vi "Example Configuration.vi"() -> ()   [LabVIEW 2010]
uses:
  C:/tf/play/labview/Tinkerforge.dll
  Tinkerforge.dll
panel:
  in  "stop":bool
  in  "uid":string="63oL6P"
  in  "port":i32=4223
  in  "host":string="localhost"
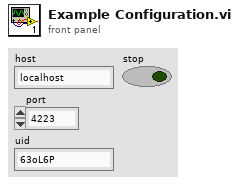
[diagram p1: front panel]
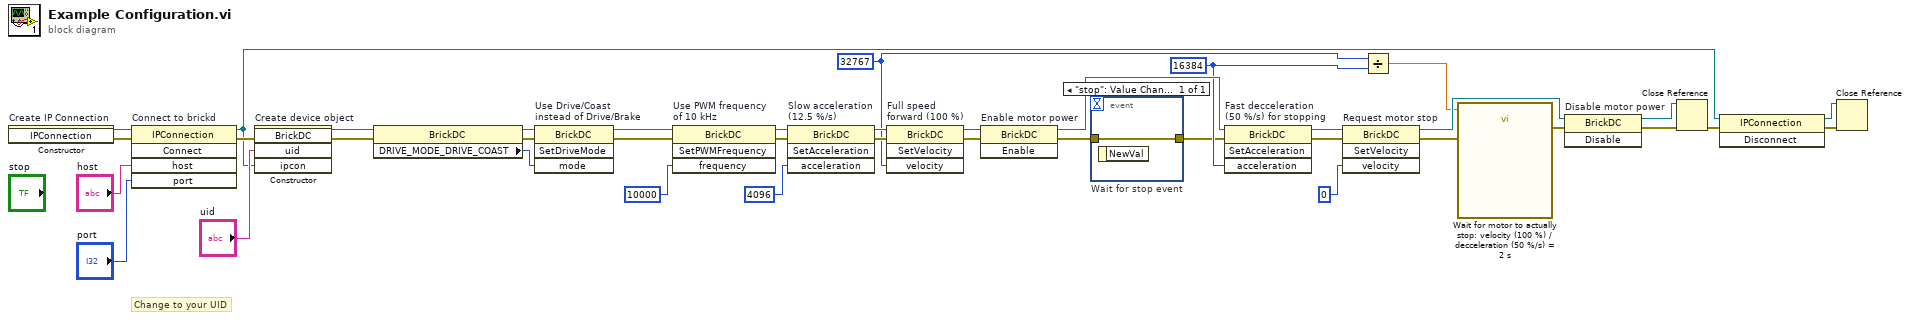
[diagram p0: block diagram]
diagram:
  w3 = 16384 ("acceleration")
  w4 = i16 32767 ("velocity")
  # "Change to your UID"
  n1 = constructor on="Create IP Connection" class="IPConnection"() -> (reference out=w39:refnum<k24>, error out=w21:errorcluster)  [unwired: 3 in, 1 out]
  n2 = invoke on="Connect to brickd" class="IPConnection" method="Connect"(reference=w39, error in=w21, "host"="host", "port"="port") -> (reference out=w32:refnum<k24>, error out=w35:errorcluster)  [unwired: 1 in, 3 out]
  n3 = constructor on="Create device object" class="BrickDC"(error in=w35, "uid"="uid", "ipcon"=w32) -> (reference out=w19:refnum<k24>, error out=w20:errorcluster)  [unwired: 2 in, 3 out]
  n4 = property class="BrickDC"(reference=w19, error in=w20) -> (reference out=w23:refnum<k24>, error out=w24:errorcluster, "DRIVE_MODE_DRIVE_COAST"=w22:u8)
  n5 = invoke on="Use Drive/Coast\ninstead of Drive/Brake" class="BrickDC" method="SetDriveMode"(reference=w23, error in=w24, "mode"=w22) -> (reference out=w18:refnum<k24>, error out=w17:errorcluster)  [unwired: 1 in, 2 out]
  n6 = invoke on="Use PWM frequency\nof 10 kHz" class="BrickDC" method="SetPWMFrequency"(reference=w18, error in=w17, "frequency"=10000 ("current")) -> (reference out=w15:refnum<k24>, error out=w16:errorcluster)  [unwired: 1 in, 2 out]
  n7 = invoke on="Slow acceleration\n(12.5 %/s)" class="BrickDC" method="SetAcceleration"(reference=w15, error in=w16, "acceleration"=4096 ("velocity")) -> (reference out=w27:refnum<k24>, error out=w28:errorcluster)  [unwired: 1 in, 2 out]
  n8 = invoke on="Full speed\nforward (100 %)" class="BrickDC" method="SetVelocity"(reference=w27, error in=w28, "velocity"=w4) -> (reference out=w25:refnum<k24>, error out=w26:errorcluster)  [unwired: 1 in, 2 out]
  n9 = invoke on="Enable motor power" class="BrickDC" method="Enable"(reference=w25, error in=w26) -> (reference out=w14:refnum<k24>, error out=w1:errorcluster)  [unwired: 1 in, 1 out]
  n10 = event "Wait for stop event" shown="[0] \"stop\": Value Change" {
    selector: _ -> [_]
    dyn-events: _ -> [_]
    timeout: _ -> [_]
    tunnel: [w40] -> w2
    tunnel: w1 -> [w40]
    event "stop": Value Change {
      n11 = event-data() -> ()  [unwired: 1 in, 1 out]
    }
  }
  n12 = invoke on="Fast decceleration\n(50 %/s) for stopping" class="BrickDC" method="SetAcceleration"(reference=w14, error in=w2, "acceleration"=w3) -> (reference out=w13:refnum<k24>, error out=w12:errorcluster)  [unwired: 1 in, 2 out]
  n13 = invoke on="Request motor stop" class="BrickDC" method="SetVelocity"(reference=w13, error in=w12, "velocity"=i16 0) -> (reference out=w6:refnum<k24>, error out=w8:errorcluster)  [unwired: 1 in, 2 out]
  n14 = Divide(x=w4, y=w3) -> (x/y=w5:dbl)
  n15 = call "Wait for motor to actually stop: velocity (100 %) / decceleration (50 %/s) = 2 s"("error in (no error)"=w8, "Delay Time (s)"=w5) -> ("error out"=w7:errorcluster)  [unwired: 9 in]
  n16 = invoke on="Disable motor power" class="BrickDC" method="Disable"(reference=w6, error in=w7) -> (reference out=w10:refnum<k24>, error out=w9:errorcluster)  [unwired: 1 in, 1 out]
  n17 = Close Reference(reference=w10, error in (no error)=w9) -> (error out=w34:errorcluster)
  n18 = invoke class="IPConnection" method="Disconnect"(reference=w32, error in=w34) -> (reference out=w31:refnum<k24>, error out=w33:errorcluster)  [unwired: 1 in, 1 out]
  n19 = Close Reference(reference=w31, error in (no error)=w33) -> ()  [unwired: 1 out]
